vi "saveSettings.vi"(11 "VI in":refnum<vi>) -> ()   [LabVIEW 2017]
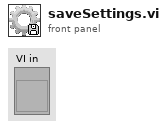
[diagram p1: front panel]
types:
  T1 = enum16{"open", "replace", "create", "open or create", "replace or create", "replace or create with confirmation"}
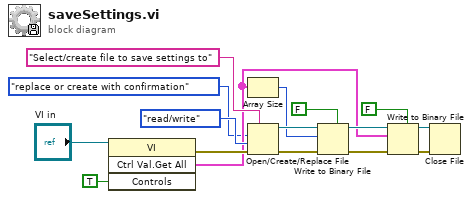
[diagram p0: block diagram]
diagram:
  n1 = invoke class="VI" method="Ctrl Val.Get All"(reference="VI in", "Controls"=TRUE) -> (error out=w13:errorcluster, "Get All Control Values Variant"=w5:cluster{"Name":string, "Variant Data":variant}[])  [unwired: 2 in, 2 out]
  n2 = Array Size(array=w5) -> (size(s)=w6:i32)
  n3 = Open/Create/Replace File(error in=w13, prompt="Select/create file to save settings to", operation (0:open)=T1."replace or create with confirmation", access (0:read/write)=enum16{"read/write", "read-only", "write-only"}."read/write") -> (refnum out=w9:refnum<file>, error out=w12:errorcluster)  [unwired: 2 in, 1 out]
  n4 = Write to Binary File(file (use dialog)=w9, data=w6, error in=w12, 5:FALSE ("prepend array or string size? (T)")) -> (refnum out=w8:refnum<file>, error out=w11:errorcluster)  [unwired: 2 in, 1 out]
  n5 = Write to Binary File(file (use dialog)=w8, data=w5, error in=w11, 5:FALSE ("prepend array or string size? (T)")) -> (refnum out=w15:refnum<file>, error out=w16:errorcluster)  [unwired: 2 in, 1 out]
  n6 = Close File(refnum=w15, error in=w16) -> ()  [unwired: 2 out]
